vi "setHPData.vi"(10 "HPData":T1 {"Responses"."ForceAndStatus" items=["OK", "IllegalFunction", "IllegalDataAddress", "IllegalDataValue", "SlaveDeviceFailure", "Acknowledge", "SlaveDeviceBusy", "NegativeAcknowledge", "MemoryParityError", "GatewayPathUnavailable", "GatewayTargetDeviceFailedToRespond"]; "Responses"."StepMotor" items=["OK", "IllegalFunction", "IllegalDataAddress", "IllegalDataValue", "SlaveDeviceFailure", "Acknowledge", "SlaveDeviceBusy", "NegativeAcknowledge", "MemoryParityError", "GatewayPathUnavailable", "GatewayTargetDeviceFailedToRespond"]}, 11 "HardPointActuator in":refnum<class "HPILC.lvclass">) -> (3 "HardPointActuator out":refnum<class "HPILC.lvclass">)   [LabVIEW 2016, in "RTHPILC.lvlib" / "HPILC.lvclass"]
uses:
  HPILC.lvclass
  DataTypes/HPData.ctl
  DataTypes/HPConstants.ctl
  DataTypes/HPCommand.ctl
  DataTypes/HPTelemetry.ctl
  DataTypes/HPResponses.ctl
  Common_RT_Modbus/DataTypes/ExceptionCodes.ctl
  DataTypes/HPTimings.ctl
  HPILC.lvclass/HPILC.ctl
  RTHPILC.lvlib
  Common_RT_Modbus/RTModbus.lvlib
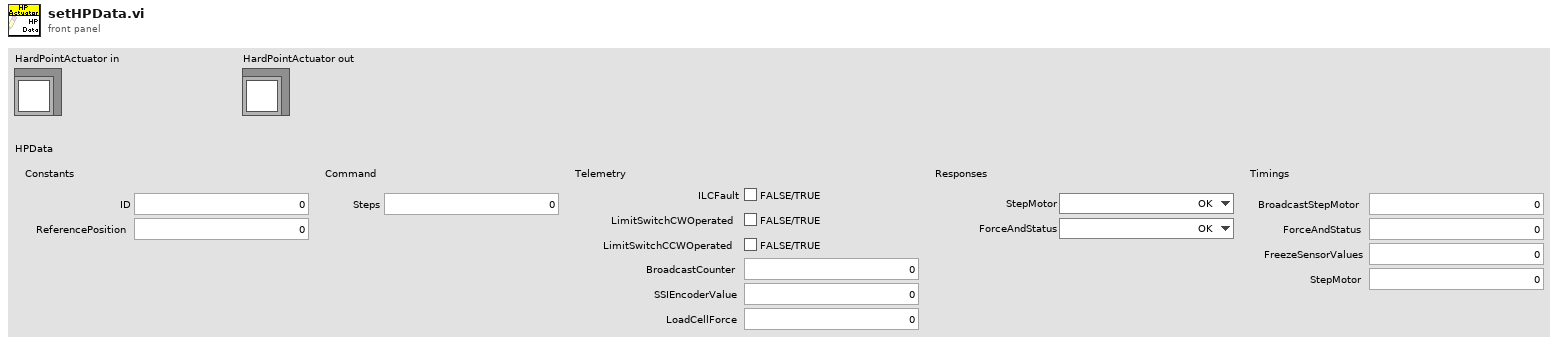
[diagram p1: front panel]
types:
  T1 = typedef "RTHPILC.lvlib/HPData.ctl" = cluster{"Constants":T2, "Command":T3, "Telemetry":T4, "Responses":T5, "Timings":T7}
  T2 = typedef "RTHPILC.lvlib/HPConstants.ctl" = cluster{"ID":i16, "ReferencePosition":i32}
  T3 = typedef "RTHPILC.lvlib/HPCommand.ctl" = cluster{"Steps":i8}
  T4 = typedef "RTHPILC.lvlib/HPTelemetry.ctl" = cluster{"ILCFault":bool, "LimitSwitchCWOperated":bool, "LimitSwitchCCWOperated":bool, "BroadcastCounter":u8, "SSIEncoderValue":i32, "LoadCellForce":sgl}
  T5 = typedef "RTHPILC.lvlib/HPResponses.ctl" = cluster{"StepMotor":T6, "ForceAndStatus":T6}
  T6 = typedef "RTModbus.lvlib/ExceptionCodes.ctl" = u16
  T7 = typedef "RTHPILC.lvlib/HPTimings.ctl" = cluster{"BroadcastStepMotor":u32, "ForceAndStatus":u32, "FreezeSensorValues":u32, "StepMotor":u32}
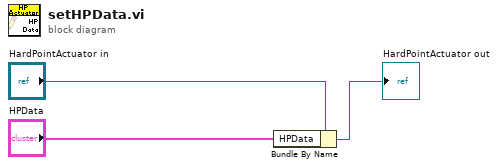
[diagram p0: block diagram]
diagram:
  n1 = Bundle By Name(cluster="HardPointActuator in", "HPData"="HPData") -> (→"HardPointActuator out":refnum<class "HPILC.lvclass">)
